vi "Vision_Left_R2.0.vi"() -> ()   [LabVIEW 2015]
uses:
  <vilib>/vision/Pattern Matching.llb/IMAQ Curve Parameters.ctl
  <vilib>/vision/Pattern Matching.llb/IMAQ Match Range Setting.ctl
panel:
  out "Current Correlation":sgl
  in  "Correlation Score Threshold":sgl
  out "New Min Score":dbl=879.6385864257812
  out "New Low Scale":dbl=38.665856552124026
  out "New high Scale":dbl=79.77148170471192
  in  "Absolute\nMinimum Score":dbl=800.0
  in  "Absolute\nMaximum Scale":dbl=300.0
  in  "Absolute\nMinimum Scale":dbl=10.0
  in  "Score Decay \nFactor":dbl=50.0
  in  "ROI_factor(Horiztonal) (4 b)":sgl=5.0
  in  "ROI_factor(vertical) (4 b)":sgl=1.5
  in  "ROI_factor(vertical) (5 b)":sgl=2.7
  in  "ROI_factor(Horiztonal) (5 b)":sgl=4.7
  in  "ROI_factor(Horiztonal) (2 b)":sgl=1.5
  in  "ROI_factor(vertical) (2 b)":sgl=2.5
  in  "Minimum Score\nSub 2":dbl=950.0
  in  "Minimum Score\nSub 3":dbl=900.0
  in  "Minimum Score\nSub 4":dbl=850.0
  in  "Minimum Score\nNormal 5":dbl=800.0
  in  "ROBOT STATE\n(fwd, bwd, neither)":i32
  out "Scale \nCushion":dbl=20.552812576293945
  in  "Score\nCushion":dbl=150.0
  in  "Default No Lock\nSetting Values":T1={"Min Scale"=20.0, "Max Scale"=170.0, "Min Score"=800.0}
  out "Next Template":T2(ring)
  in  "4 / 3\nTransition Scale":sgl=85.0
  in  "5 / 4\nTransition Scale":sgl=60.0
  in  "3 / 2\nTransition Scale":sgl=100.0
  in  "Avg Scale - Last":dbl=59.21866912841797
  in  "Avg Score - Last":dbl=954.6385864257812
  in  "Max Window\n for Avg":u8=5
  in  "Valid Treshold\nfor Lock":i16=3
  out "Current  Score":sgl=951.2561
  out "Current  Scale":sgl=59.269463
  out "Current Valid?":bool
  out "Beacon - Scales":sgl[](array[numeric])=[0.0, 59.087868, 59.67315, 57.828133, 55.61106]
  out "beacon - Scores":sgl[](array[numeric])=[0.0, 997.01117, 999.39996, 999.517, 998.72253]
  out "Beacons Found":bool[](array[boolean])=[FALSE, TRUE, TRUE, TRUE, TRUE]
  in  "Horiztonall Beacon \nCushion (pixels)":sgl=20.0
  in  "Sub - 4 - FIle Path":path=path "/home/lvuser/natinst/bin/BeaconTemplates/4_beacons_left.png"
  in  "Sub - 2 File Path":path=path "/home/lvuser/natinst/bin/BeaconTemplates/2_beacons_left.png"
  in  "Sub Beacon Template File Path - ARRAY":path[](array[path])=[path "/home/lvuser/natinst/bin/BeaconTemplates/Sub1.png", path "/home/lvuser/natinst/bin/BeaconTemplates/Sub2.png", path "/home/lvuser/natinst/bin/BeaconTemplates/Sub3.png", path "/home/lvuser/natinst/bin/BeaconTemplates/Sub4.png", path "/home/lvuser/natinst/bin/BeaconTemplates/Sub5.png"]
  in  "Sub - 3 - FIle Path":path=path "/home/lvuser/natinst/bin/BeaconTemplates/3_beacons_left.png"
  in  "Normal - 5 - File Path":path=path "/home/lvuser/natinst/bin/BeaconTemplates/5_beacons.png"
  out "Tracking Info":T3={"Tracking Coordinates"={"X"=154.8973846435547, "Y"=87.84130859375}, "Current Valid"=TRUE, "Current State - Out"=enum."Sub - 2", "Setting Values"={"Min Score"=950.0, "Min Scale"=103.51155548095704, "Max Scale"=214.8787582397461}}
  out "Current Template":T2(ring)
  in  "Initial Template":T2(ring)
  out "dT":u32=1105
  out "Avg Scale":dbl=159.2824279785156
  out "Avg Score":dbl=995.22490234375
  out "Current Search Settings":T6={"Curve Parameters"={"Extraction Mode"=1, "Edge Threshold"=150, "Edge Filter Size"=0, "Min Length"=15, "Row Search Step Size"=10, "Col Search Step Size"=10, "Max Endpoint Gap"=2, "Closed"=TRUE, "Subpixel"=TRUE}, "Match Mode"={"Rotation"=FALSE, "Scale"=TRUE, "Occlusion"=TRUE, "Reserved"=FALSE, "Reserved"=FALSE, "Reserved"=FALSE}, "Range Settings"=[{"Match Constraints"=0, "Min"=-2.0, "Max"=2.0}, {"Match Constraints"=1, "Min"=103.59702987670897, "Max"=214.96782608032225}, {"Match Constraints"=2, "Min"=0.0, "Max"=20.0}], "Number of Matches"=1, "Minimum Match Score"=950.0, "SubPixel Accuracy"=TRUE, "Adv. Geometric Match Options 2"=[{"Setup Data Item"=20, "Item Value"=0.0}, {"Setup Data Item"=22, "Item Value"=1.0}]} {"Curve Parameters"."Extraction Mode" items=["Normal", "Uniform Regions"]; "Curve Parameters"."Edge Filter Size" items=["Fine", "Normal", "Contour Tracing"]; "Curve Parameters"."Max Endpoint Gap" min=0; "Curve Parameters"."Col Search Step Size" min=1 max=255 step=1; "Curve Parameters"."Row Search Step Size" min=1 max=255 step=1; "Curve Parameters"."Min Length" min=0; "Curve Parameters"."Edge Threshold" min=1 max=350 step=1; "Range Settings"."Max" format="%.2f"; "Range Settings"."Min" format="%.2f"; "Range Settings"."Match Constraints" items=["Rotation Angle (degrees)", "Scale Factor (%)", "Occlusion (%)"]}
  out "Valid Scale History":dbl[](array[numeric])=[159.54193115234375, 159.0799560546875, 159.38912963867188, 159.05020141601562, 159.35092163085938, 159.10557556152344, 159.3151092529297, 159.3177947998047, 159.0937957763672, 159.64999389648438, 159.23023986816406, 159.07296752929688, 159.37905883789062, 156.36964416503906, 151.1900634765625, 132.892578125, 119.50423431396484, 108.0020523071289, 99.8529052734375, 93.15778350830078] format="%#_13g"
  out "Valid Score History":dbl[](array[numeric])=[995.82177734375, 997.0046997070312, 997.0046997070312, 997.0046997070312, 989.2886352539062, 997.0046997070312, 997.0046997070312, 996.4745483398438, 996.4745483398438, 995.4120483398438, 996.692138671875, 996.692138671875, 996.692138671875, 996.337890625, 998.2847290039062, 996.9906616210938, 1000.0, 999.7824096679688, 999.7824096679688, 999.7824096679688] format="%#_13g"
  out "Valid Beacon History - in":bool[](array[boolean])=[TRUE, TRUE, TRUE, TRUE, TRUE, TRUE, TRUE, TRUE, TRUE, TRUE, TRUE, TRUE, TRUE, TRUE, TRUE, TRUE, TRUE, TRUE, TRUE, TRUE]
  out "Startup Flag":bool
  out "Lock Status":bool
  out "Y Coordinates":sgl[](array[numeric])=[100.60873, 0.0, 0.0, 0.0, 0.0]
  out "X Coordinates":sgl[](array[numeric])=[108.138504, 0.0, 0.0, 0.0, 0.0]
  out "Right Image out":T7(plugin-control)
  in  "History Size":i32=20
  in  "INITIAL Search Settings":T6={"Curve Parameters"={"Extraction Mode"=1, "Edge Threshold"=150, "Edge Filter Size"=0, "Min Length"=15, "Row Search Step Size"=10, "Col Search Step Size"=10, "Max Endpoint Gap"=2, "Closed"=TRUE, "Subpixel"=TRUE}, "Match Mode"={"Rotation"=FALSE, "Scale"=TRUE, "Occlusion"=TRUE, "Reserved"=FALSE, "Reserved"=FALSE, "Reserved"=FALSE}, "Range Settings"=[{"Match Constraints"=0, "Min"=-2.0, "Max"=2.0}, {"Match Constraints"=1, "Min"=25.0, "Max"=100.0}, {"Match Constraints"=2, "Min"=0.0, "Max"=20.0}], "Number of Matches"=1, "Minimum Match Score"=800.0, "SubPixel Accuracy"=TRUE, "Adv. Geometric Match Options 2"=[{"Setup Data Item"=20, "Item Value"=0.0}, {"Setup Data Item"=22, "Item Value"=1.0}]} {"Curve Parameters"."Extraction Mode" items=["Normal", "Uniform Regions"]; "Curve Parameters"."Edge Filter Size" items=["Fine", "Normal", "Contour Tracing"]; "Curve Parameters"."Max Endpoint Gap" min=0; "Curve Parameters"."Col Search Step Size" min=1 max=255 step=1; "Curve Parameters"."Row Search Step Size" min=1 max=255 step=1; "Curve Parameters"."Min Length" min=0; "Curve Parameters"."Edge Threshold" min=1 max=350 step=1; "Range Settings"."Max" format="%.2f"; "Range Settings"."Min" format="%.2f"; "Range Settings"."Match Constraints" items=["Rotation Angle (degrees)", "Scale Factor (%)", "Occlusion (%)"]; "Adv. Geometric Match Options 2"."Setup Data Item" items=["Curve Extraction Mode", "Curve Edge Threshold", "Curve Edge Filter Size", "Min Curve Length", "Curve Row Search Step Size", "Curve Col Search Step Size", "Curve Max Endpoint Gap", "Extract Closed Curves", "Enable Subpixel Curve Extraction", "Enable Correlation Score", "Enable Subpixel Accuracy", "Subpixel Iterations", "Subpixel Tolerance", "Initial Match List Length", "Enable Target Template Curve Score", "Min Match Separation Distance", "Min Match Separation Angle", "Min Match Separation Scale", "Max Match Overlap", "Enable Coarse Result", "Enable Calibration Support", "Enable Contrast Reversal", "Search Strategy", "Refinement Match Factor", "Subpixel Match Factor"]}
  # "TEMPLATE FILE PATHS"
  # "Current Match Values"
  # "Range"
  # "Range"
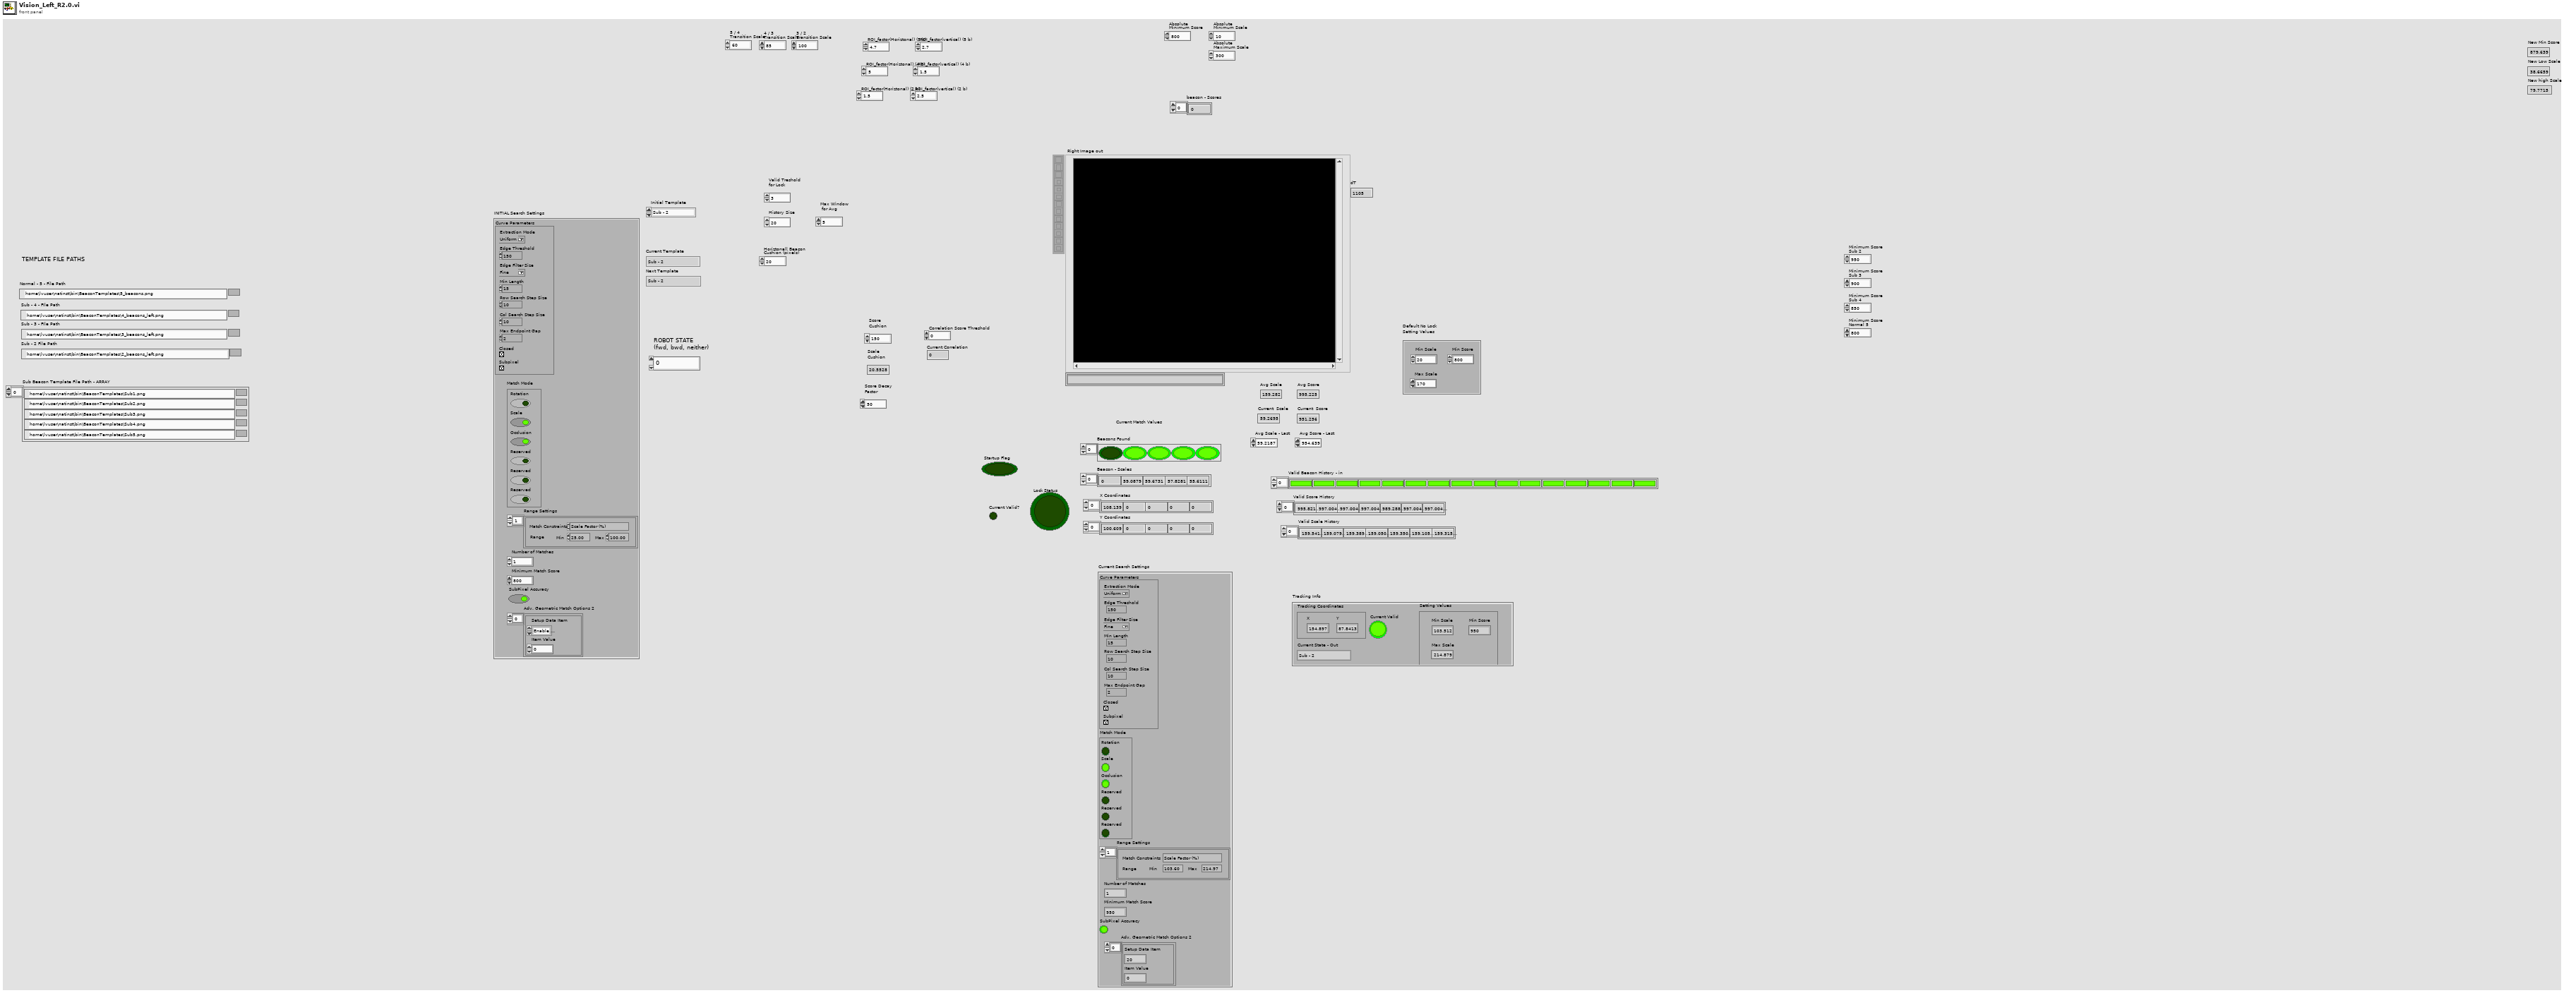
[diagram p1: front panel]
types:
  T1 = cluster{"Min Scale":dbl, "Max Scale":dbl, "Min Score":dbl}
  T2 = enum16{"Sub - 2", "Sub - 3", "Sub - 4", "Normal - 5"}
  T3 = cluster{"Tracking Coordinates":cluster{"X":dbl, "Y":dbl}, "Current Valid":bool, "Current State - Out":enum16{"Sub - 2", "Sub - 3", "Sub - 4", "Normal - 5"}, "Setting Values":cluster{"Min Score":dbl, "Min Scale":dbl, "Max Scale":dbl}}
  T4 = typedef "IMAQ Curve Parameters.ctl" = cluster{"Extraction Mode":u32, "Edge Threshold":i32, "Edge Filter Size":u32, "Min Length":i32, "Row Search Step Size":i32, "Col Search Step Size":i32, "Max Endpoint Gap":i32, "Closed":bool, "Subpixel":bool}
  T5 = typedef "IMAQ Match Range Setting.ctl" = cluster{"Match Constraints":u32, "Min":dbl, "Max":dbl}
  T6 = cluster{"Curve Parameters":T4, "Match Mode":cluster{"Rotation":bool, "Scale":bool, "Occlusion":bool, "Reserved":bool, "Reserved":bool, "Reserved":bool}, "Range Settings":T5[], "Number of Matches":i32, "Minimum Match Score":sgl, "SubPixel Accuracy":bool, "Adv. Geometric Match Options 2":cluster{"Setup Data Item":u16, "Item Value":dbl}[]}
  T7 = typedef "IMAQ Image.ctl" = refnum<image>
  T8 = typedef "Image Type" = u32
  T9 = typedef "ROI Descriptor" = cluster{"Global Rectangle":i32[], "Contours":cluster{"ID":enum32{"External", "Internal"}, "Type":u32, "Coordinates":i32[]}[]}
  T10 = typedef "IMAQ GM Match Report.ctl" = cluster{"Position":cluster{"x":sgl, "y":sgl}, "Angle":sgl, "Scale":sgl, "Score":sgl, "Bounding Box":cluster{"x":sgl, "y":sgl}[], "Contrast Reversed":bool, "Occlusion %":sgl, "Template Target Curve Score":sgl, "Target Template Curve Score":sgl, "Correlation Score":sgl}
  T11 = cluster{"Matches (Geometric Matching 1)[0]":T10, "Matches (Geometric Matching 1)[1]":T10, "Matches (Geometric Matching 1)[2]":T10, "Matches (Geometric Matching 1)[3]":T10, "Matches (Geometric Matching 1)[4]":T10, "Matches (Geometric Matching 1)[5]":T10, "Matches (Geometric Matching 1)[6]":T10, "Matches (Geometric Matching 1)[7]":T10, "Matches (Geometric Matching 1)[8]":T10}
  T12 = cluster{"Bounding Box[0]":cluster{"x":sgl, "y":sgl}, "Bounding Box[1]":cluster{"x":sgl, "y":sgl}, "Bounding Box[2]":cluster{"x":sgl, "y":sgl}, "Bounding Box[3]":cluster{"x":sgl, "y":sgl}, "Bounding Box[4]":cluster{"x":sgl, "y":sgl}, "Bounding Box[5]":cluster{"x":sgl, "y":sgl}, "Bounding Box[6]":cluster{"x":sgl, "y":sgl}, "Bounding Box[7]":cluster{"x":sgl, "y":sgl}, "Bounding Box[8]":cluster{"x":sgl, "y":sgl}}
  T13 = cluster{"Tracking Coordinates":cluster{"X":dbl, "Y":dbl}, "Current Valid":bool, "Current State - Out":enum16{"Sub - 2", "Sub - 3", "Sub - 4", "Normal - 5"}, "Setting Values":cluster{"Min Scale":dbl, "Max Scale":dbl, "Min Score":dbl}}
  T14 = typedef "IMAQ Rectangle" = cluster{"Left":i32, "Top":i32, "Right":i32, "Bottom":i32, "Rotation":dbl}
  T15 = cluster{"Minimum Score\nNormal 5":dbl, "Min":dbl, "Max":dbl}
  T16 = cluster{"Position":cluster{"x":dbl, "y":dbl}, bool, "Next Template":enum16{"Sub - 2", "Sub - 3", "Sub - 4", "Normal - 5"}, cluster{"Minimum Score\nNormal 5":dbl, "Min":dbl, "Max":dbl}}
  T17 = cluster{"Position":cluster{"x":dbl, "y":dbl}, bool, "Current Template":enum16{"Sub - 2", "Sub - 3", "Sub - 4", "Normal - 5"}, cluster{"Minimum Score\nNormal 5":dbl, "Min":dbl, "Max":dbl}}
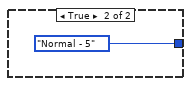
[diagram p3: hidden frame]
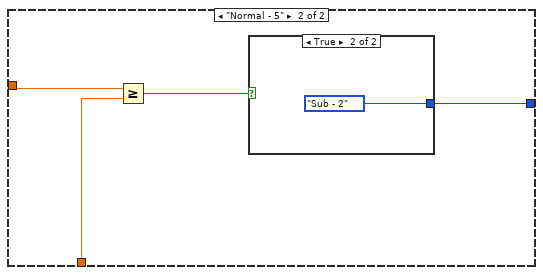
[diagram p4: hidden frame]
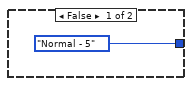
[diagram p5: hidden frame]
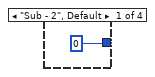
[diagram p7: hidden frame]
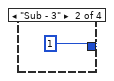
[diagram p8: hidden frame]
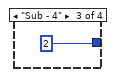
[diagram p9: hidden frame]
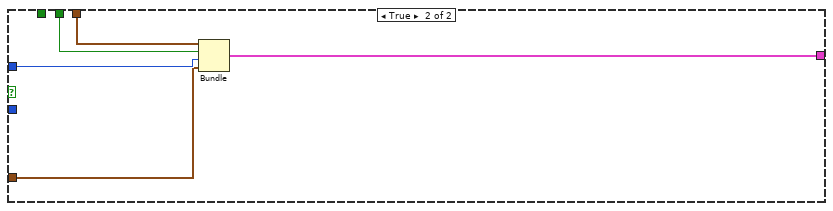
[diagram p10: hidden frame]
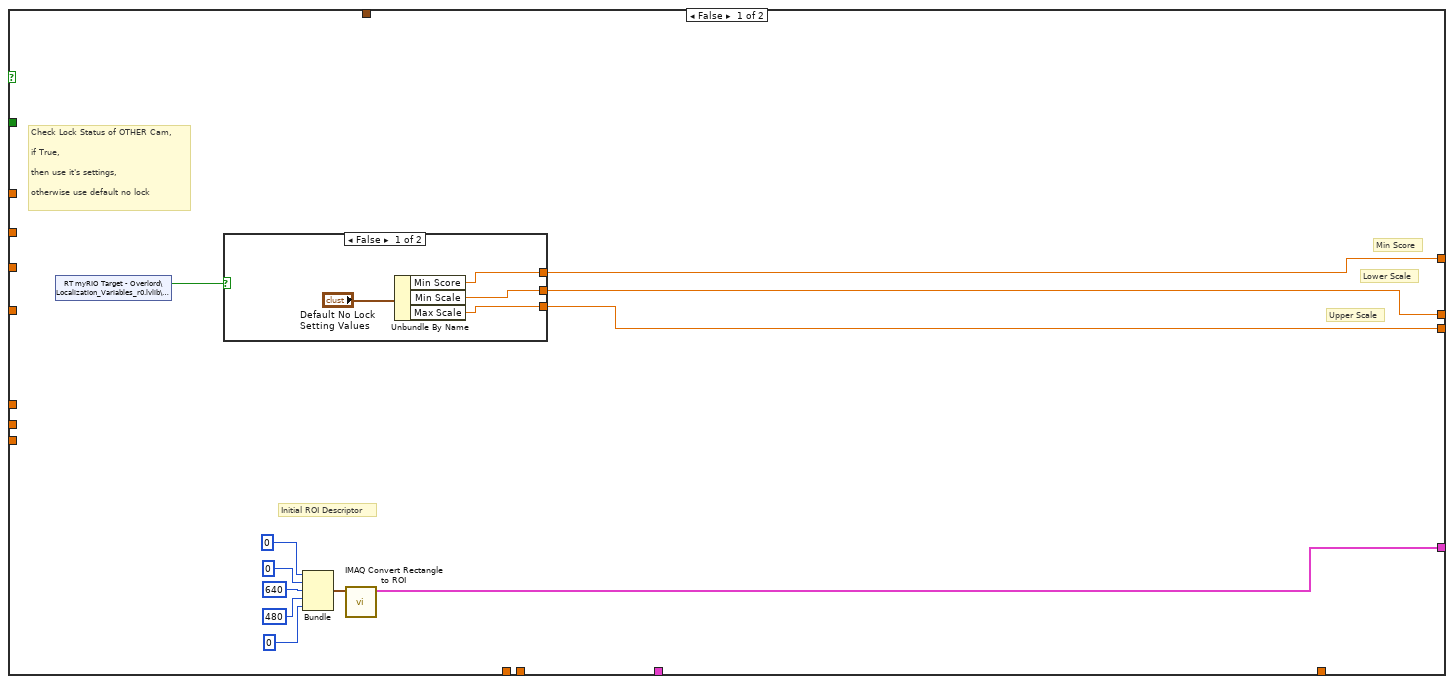
[diagram p13: hidden frame]
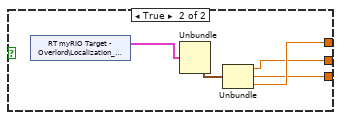
[diagram p14: hidden frame]
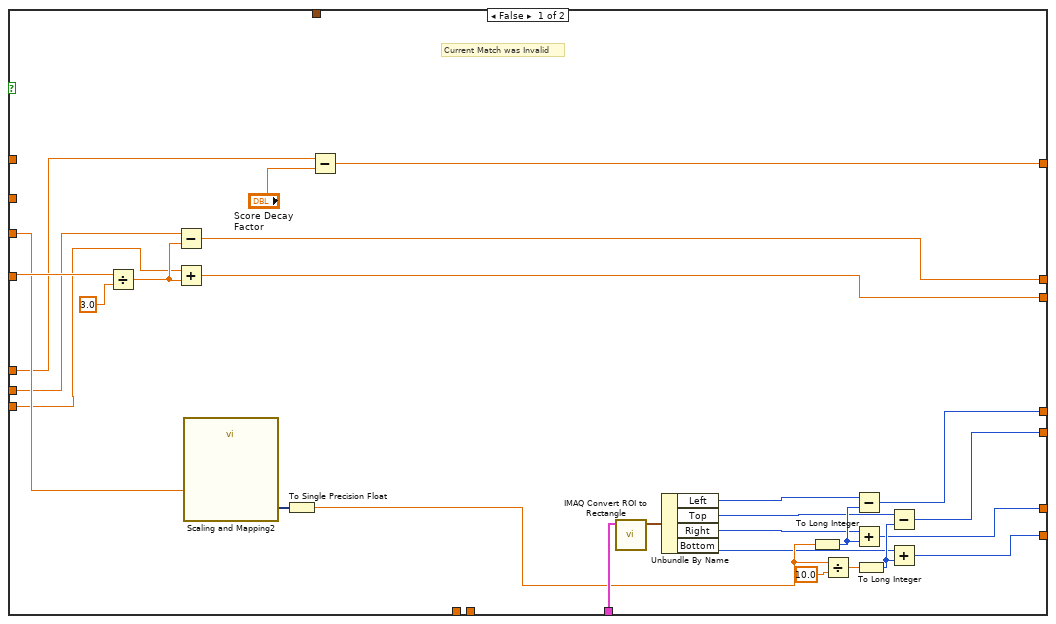
[diagram p15: hidden frame]
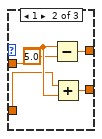
[diagram p16: hidden frame]
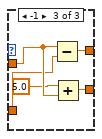
[diagram p17: hidden frame]
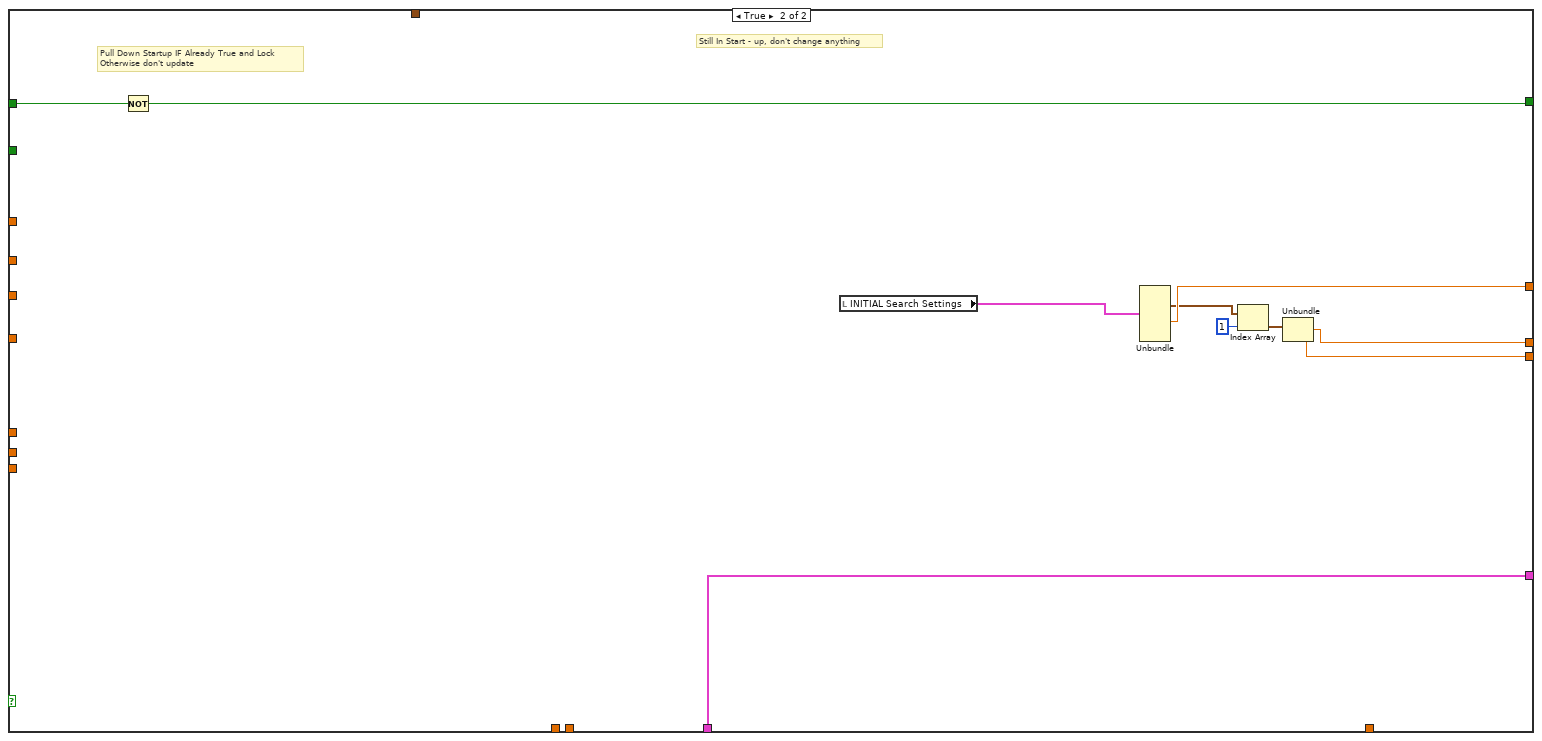
[diagram p18: hidden frame]
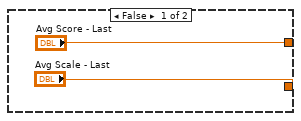
[diagram p19: hidden frame]
diagram:
  n1 = flat-sequence {
    tunnel: [w24] -> w12
    tunnel: ["INITIAL Search Settings"] -> w11
    tunnel: ["Initial Template"] -> w10
    tunnel: [TRUE] -> w9
    tunnel: [w21] -> w8
    tunnel: [w20] -> w7
    tunnel: [w19] -> w6
    tunnel: [w18] -> w5
    tunnel: [w17] -> w4
    tunnel: ["History Size"] -> w3
    tunnel: [750.0] -> w2
    tunnel: [100.0] -> w1
    tunnel: w12 -> [w46]
    tunnel: w11 -> [w45]
    tunnel: w10 -> [w44]
    tunnel: w9 -> [w43]
    tunnel: w8 -> [w39]
    tunnel: w7 -> [w36]
    tunnel: w6 -> [w42]
    tunnel: w5 -> [w41]
    tunnel: w4 -> [w40]
    tunnel: w3 -> [w38]
    tunnel: w2 -> [_]
    tunnel: w1 -> [_]
    frame #0 {
      w31 = T8 0 items=["Grayscale (U8)", "Grayscale (I16)", "Grayscale (SGL)", "Complex (CSG)", "RGB (U32)", "HSL (U32)", "RGB (U64)", "Grayscale (U16)"] ("Image Type")
      # "avg start scale"
      # "Score History"
      # "Scale History"
      # "Valid Match History\n(main beacon)"
      # "Template State"
      # "Search Parameters"
      # "StartUp = True"
      # "Initial ROI Descriptor"
      # "INITIALIZE"
      n2 = Bundle(0, 0, 640, 480, 0) -> (w30:cluster{i32, i32, i32, i32, i32})  [unwired: 1 in]
      n3 = call "IMAQ Convert Rectangle to ROI"("Rectangle"=w30) -> ("ROI Descriptor"=w24:T9)  [unwired: 8 in, 1 out]
      n4 = call "IMAQ Create"("Image Name"="Left_Image", "Image Type"=w31) -> ("New Image"=w21:T7, "error out"=w20:errorcluster)  [unwired: 3 in]
      n5 = Initialize Array(FALSE, "History Size") -> (w19:bool[])
      n6 = Initialize Array(0.0, "History Size") -> (w17:dbl[])
      n7 = Initialize Array(0.0, "History Size") -> (w18:dbl[])
    }
    frame #1 {
      # "Avg Scale"
      # "Avg Score"
      # "Score History"
      # "Scale History"
      # "Valid Match History\n(main beacon)"
      # "Sub Beacon Search Array"
      # "StartUp = True"
      # "Template State"
      # "Search Parameters"
      # "ROI"
      n8 = call "Tick Count"() -> ("Tick Count(mSec)"=w37:u32)
      n9 = while {
        shift-right: [w58] -> _
        shift-left: w46 -> [w65]
        shift-right: [w59] -> _
        shift-left: w45 -> [w66]
        shift-right: [w56] -> _
        shift-left: w44 -> [w74]
        shift-right: [w62] -> _
        shift-left: w43 -> [w64]
        shift-right: [w51] -> _
        shift-left: w42 -> [w52]
        shift-right: [w49] -> _
        shift-left: w41 -> [w50]
        shift-right: [w47] -> _
        shift-left: w40 -> [w48]
        shift-right: [w54] -> _
        shift-left: w39 -> [w67]
        tunnel: w38 -> [w72]
        shift-right: [w70] -> _
        shift-left: w37 -> [w71]
        tunnel: w36 -> [w53]
        stop <- FALSE stop-if-true
        n10 = call "Tick Count2"() -> ("Tick Count(mSec)"=w70:u32)
        n11 = Subtract(x=w70, y=w71) -> (x-y=→"dT":u32)
        n12 = flat-sequence {
          tunnel: [w81] -> w75
          tunnel: [w80] -> w73
          tunnel: [w79] -> w61
          tunnel: [w78] -> w68
          tunnel: w67 -> [w78]
          tunnel: [w78] -> w54
          tunnel: w53 -> [w77]
          tunnel: w75 -> [w195]
          tunnel: w74 -> [w95]
          tunnel: w73 -> [w100]
          tunnel: w52 -> [w176]
          tunnel: w50 -> [w175]
          tunnel: w48 -> [w174]
          tunnel: w72 -> [_]
          tunnel: w68 -> [w189]
          tunnel: w66 -> [w119]
          tunnel: w65 -> [w142]
          tunnel: w64 -> [w159]
          tunnel: [w118] -> w63
          tunnel: [w114] -> w62
          tunnel: w61 -> [w103]
          tunnel: [w103] -> w60
          tunnel: [w102] -> w57
          tunnel: [w101] -> w55
          tunnel: [w98] -> w51
          tunnel: [w97] -> w49
          tunnel: [w96] -> w47
          tunnel: w63 -> [w589]
          tunnel: w60 -> [w590]
          tunnel: [w589] -> w59
          tunnel: [w588] -> w58
          tunnel: w57 -> [w588]
          tunnel: [w587] -> w56
          tunnel: w55 -> [w587]
          frame #0 {
            # "Aquire Image"
            n13 = shared-variable "RT myRIO Target - Overlord\\Localization_Variables_r0.lvlib\\Left Servo Angle_Current"() -> (w79:dbl)  [unwired: 1 in, 1 out]
            n14 = call "Camera Acquisition"("error in"=w77) -> ("Image Out"=w81:T7, "error out"=w80:errorcluster)  [unwired: 24 in, 1 out]
          }
          frame #1 {
            w122 = u32 1 ("index")
            # "Current Template"
            # "Check if Next Template == Current TEmplate"
            # "Update Tracking Coordinates"
            # "Next Settings"
            # "Current Settings"
            # "Current Min\n& Max Scale"
            # "Scale"
            # "Min Score"
            # "Lower Scale"
            # "Upper Scale"
            # "Min Score out"
            # "Choose ROI Factor based on Next State"
            # "Avg Scale"
            # "Avg Score"
            # "StartUp Flag"
            # "Current Valid"
            # "image Lock"
            # "Update Search Settings"
            # "Image Lock?"
            # "Update Template"
            # "Score History"
            # "Min Required to use avarage"
            # "Scale History"
            # "History Size"
            # "Calculate Average Score/Scale"
            # "****# of previous in history that must be true\nin order for position to be considered \"locked\""
            # "Scale History"
            # "Score History"
            # "Valid History"
            # "Update History Data"
            # "1 Match FOund?"
            # "# of Sub Beacons"
            # "Sub Beacons to Search For"
            # "# Sub Beacons to Find in\norder to be valid"
            # "Template Filepath"
            # "Select Current Template Config"
            # "Pattern Match to Current Template"
            # "Apply FIltering"
            n15 = call "Camera - Filtering"("Image In"=w195, "Image Dst"=w189, "error in"=w100) -> ("Image Out"=w190:T7, "error out"=w99:errorcluster)  [unwired: 23 in]
            n16 = case shown="\"Normal - 5\"" w95 {
              tunnel: "Normal - 5 - File Path" -> [_ _ _ w586]
              tunnel: "Sub - 4 - FIle Path" -> [_ _ w581 _]
              tunnel: "Sub - 3 - FIle Path" -> [_ w575 _ _]
              tunnel: "Sub - 2 File Path" -> [w569 _ _ _]
              tunnel: [w569 w575 w581 w586] -> w188
              tunnel: [1 2 3 3] -> w178
              tunnel: [w567 w572 w578 w583] -> w183
              tunnel: [sgl 2.0 sgl 3.0 sgl 4.0 sgl 5.0] -> w184
              frame "Sub - 2", Default {
                w565 = FALSE
                w566 = TRUE
                n17 = Build Array(w566, w566, w565, w565, w565) -> (w567:bool[])
              }
              frame "Sub - 3" {
                w571 = FALSE
                w573 = TRUE
                n18 = Build Array(w573, w573, w573, w571, w571) -> (w572:bool[])
              }
              frame "Sub - 4" {
                w579 = TRUE
                n19 = Build Array(w579, w579, w579, w579, FALSE) -> (w578:bool[])
              }
              frame "Normal - 5" {
                (unwired) FALSE
                w584 = TRUE
                n20 = Build Array(w584, w584, w584, w584, w584) -> (w583:bool[])
              }
            }
            n21 = call "Geometric Pattern Matching"("Image In"=w190, "Image Dst"=w189, "ROI Descriptor (Geometric Matching 1)"=w142, "Settings (Geometric Matching 1)"=w119, "Template File Path (Geometric Matching 1)"=w188, "error in"=w99) -> ("Image Out"=w185:T7, "Matches (Geometric Matching 1)"=w86:T10[], "Number of Matches (Geometric Matching 1)"=w187:i32, "error out"=w182:errorcluster)  [unwired: 18 in]
            n22 = Array To Cluster(array=w86) -> (cluster=w87:T11)
            n23 = Unbundle By Name(w87) -> ("Matches (Geometric Matching 1)[0].Correlation Score"=w85:sgl)
            "Current Correlation" <- w85
            n24 = Equal?(x=w187, y=1) -> (x = y?=w89:bool)
            n25 = Greater?(x=w85, y="Correlation Score Threshold") -> (0:w88:bool)
            n26 = And(x=w89, y=w88) -> (x .and. y?=w90:bool)
            n27 = case shown="True" w90 {
              tunnel: w86 -> [_ w512]
              tunnel: w185 -> [w468 w491]
              tunnel: w184 -> [_ w506]
              tunnel: w183 -> [_ w493]
              tunnel: w182 -> [_ w490]
              tunnel: w119 -> [_ w488]
              tunnel: [w473 w486] -> w107
              tunnel: [w472 w485] -> w106
              tunnel: [w472 w484] -> w105
              tunnel: [w472 w483] -> w104
              tunnel: [w472 w482] -> w179
              tunnel: [w471 w481] -> w173
              tunnel: [w471 w480] -> w172
              tunnel: [w468 w479] -> w117
              tunnel: [w469 w478] -> w82
              frame False {
                w470 = 0.0
                w471 = sgl 0.0 ("Scale")
                n28 = Bundle(w470, w470) -> (w469:cluster{dbl, dbl})  [unwired: 1 in]
                n29 = Initialize Array(FALSE, 5 ("dimension size")) -> (w473:bool[])
                n30 = Initialize Array(0.0, 5 ("dimension size")) -> (w472:dbl[])
              }
              frame True {
                # "Build ROI for Individual Beacons Based on Main Bounding Box"
                # "Starting X Lower Bound"
                # "Beacons to Search For"
                # "Length of\nIndividual Beacon ROI"
                # "Length of Bounding Box"
                # "Draw Bounding Box on Display Image"
                n31 = Array To Cluster(array=w512) -> (cluster=w513:T11)
                n32 = Unbundle By Name(w513) -> ("Matches (Geometric Matching 1)[0].Position"=w478:cluster{"x":sgl, "y":sgl}, "Matches (Geometric Matching 1)[0].Bounding Box"=w510:cluster{"x":sgl, "y":sgl}[], "Matches (Geometric Matching 1)[0].Scale"=w481:sgl, "Matches (Geometric Matching 1)[0].Score"=w480:sgl)
                n33 = Array To Cluster(array=w510) -> (cluster=w511:T12)
                n34 = Unbundle By Name(w511) -> ("Bounding Box[0].x"=w504:sgl, "Bounding Box[0].y"=w500:sgl, "Bounding Box[2].x"=w507:sgl, "Bounding Box[2].y"=w499:sgl)
                n35 = Bundle("x"=w504, "y"=w500, "x"=w507, "y"=w499) -> (w509:cluster{"x":sgl, "y":sgl, "x":sgl, "y":sgl})  [unwired: 1 in]
                n36 = call "IMAQ Overlay Rectangle"("Rectangle"=w509, "Image"=w491) -> ("Image Out"=w487:T7)  [unwired: 8 in, 1 out]
                n37 = Subtract(x=w507, y=w504) -> (x-y=w508:sgl)
                n38 = Divide(x=w508, y=w506) -> (x/y=w505:sgl)
                n39 = Multiply(x="Horiztonall Beacon \nCushion (pixels)", y=w481) -> (x*y=w501:sgl)
                n40 = Divide(x=w501, y=sgl 100.0) -> (x/y=w496:sgl)
                n41 = Subtract(x=w500, y=w496) -> (x-y=w498:sgl)
                n42 = Add(x=w499, y=w496) -> (x+y=w497:sgl)
                n43 = for {
                  N: 5 -> [_]
                  tunnel: w493 -> [w559] mode=indexing
                  shift-right: [w553] -> _
                  shift-left: w504 -> [w558]
                  tunnel: w505 -> [w557]
                  tunnel: w498 -> [w550]
                  tunnel: w497 -> [w549]
                  tunnel: [w556] -> w492 mode=indexing
                  tunnel: w496 -> [w551]
                  # "Divide Bounding Box"
                  # "Upper Bound of Current is\nLower Bound for Next"
                  n44 = case shown="True" w559 {
                    tunnel: w558 -> [w560 w561]
                    tunnel: w557 -> [_ w563]
                    tunnel: [w560 w562] -> w553
                    tunnel: [w560 w561] -> w555
                    frame False {
                      # "Don't Care"
                    }
                    frame True {
                      # "X Lower Bound"
                      n45 = Add(x=w561, y=w563) -> (x+y=w562:sgl)
                    }
                  }
                  n46 = Subtract(x=w555, y=w551) -> (x-y=w554:sgl)
                  n47 = Add(x=w553, y=w551) -> (x+y=w552:sgl)
                  n48 = call "Bound_RO_R_R0I.vi"("Bottom Right - Y"=w549, "Right - X"=w552, "Top Left - Y"=w550, "Top  Left - x"=w554) -> ("ROI Descriptor"=w556:T9)  [unwired: 7 in]
                }
                n49 = for {
                  N: 5 -> [_]
                  tunnel: w491 -> [w526]
                  tunnel: w490 -> [w525]
                  tunnel: w492 -> [w518] mode=indexing
                  tunnel: "Sub Beacon Template File Path - ARRAY" -> [w524] mode=indexing
                  tunnel: [w523] -> w485 mode=indexing
                  tunnel: [w522] -> w484 mode=indexing
                  tunnel: [w521] -> w486 mode=indexing
                  tunnel: w493 -> [w520] mode=indexing
                  tunnel: w488 -> [w519]
                  shift-right: [w516] -> w479
                  shift-left: w487 -> [w517]
                  tunnel: [w515] -> w483 mode=indexing
                  tunnel: [w514] -> w482 mode=indexing
                  n50 = case shown="True" w520 {
                    tunnel: w526 -> [_ w541]
                    tunnel: w525 -> [_ w540]
                    tunnel: w518 -> [_ w539]
                    tunnel: w524 -> [_ w538]
                    tunnel: [w527 w534] -> w523
                    tunnel: [w527 w533] -> w522
                    tunnel: [FALSE w532] -> w521
                    tunnel: w519 -> [_ w531]
                    tunnel: [w527 w530] -> w515
                    tunnel: [w527 w529] -> w514
                    frame False {
                      w527 = sgl 0.0 ("x")
                    }
                    frame True {
                      n51 = call "Sub Beacon Pattern Match"("Image In"=w541, "ROI Descriptor (Geometric Matching 1)"=w539, "Settings (Geometric Matching 1)"=w531, "Template File Path (Geometric Matching 1)"=w538, "error in"=w540) -> ("Matches (Geometric Matching 1)"=w535:T10[], "Number of Matches (Geometric Matching 1)"=w536:i32)  [unwired: 19 in, 2 out]
                      n52 = Equal?(x=w536, y=1) -> (x = y?=w532:bool)
                      n53 = case shown="True" w532 {
                        tunnel: w535 -> [_ w547]
                        tunnel: [w542 w546] -> w534
                        tunnel: [w542 w545] -> w533
                        tunnel: [w542 w544] -> w530
                        tunnel: [w542 w543] -> w529
                        frame False {
                          w542 = sgl 0.0 ("x")
                        }
                        frame True {
                          n54 = Array To Cluster(array=w547) -> (cluster=w548:T11)
                          n55 = Unbundle By Name(w548) -> ("Matches (Geometric Matching 1)[0].Position.x"=w546:sgl, "Matches (Geometric Matching 1)[0].Position.y"=w545:sgl, "Matches (Geometric Matching 1)[0].Scale"=w544:sgl, "Matches (Geometric Matching 1)[0].Score"=w543:sgl)
                        }
                      }
                    }
                  }
                  n56 = call "IMAQ Overlay ROI"("ROI Descriptor"=w518, "Image"=w517) -> ("Image Out"=w516:T7)  [unwired: 8 in, 1 out]
                }
              }
            }
            "Beacons Found" <- w107
            "X Coordinates" <- w106
            "Y Coordinates" <- w105
            "Beacon - Scales" <- w104
            "beacon - Scores" <- w179
            "Current  Scale" <- w173
            "Current  Score" <- w172
            n57 = shared-variable "RT myRIO Target - Overlord\\Localization_Variables_r0.lvlib\\LEFT_BEACON_BOOL_array"(w107) -> ()  [unwired: 1 in, 1 out]
            n58 = shared-variable "RT myRIO Target - Overlord\\Localization_Variables_r0.lvlib\\LEFT_BEACON_X_array"(w106) -> ()  [unwired: 1 in, 1 out]
            n59 = shared-variable "RT myRIO Target - Overlord\\Localization_Variables_r0.lvlib\\LEFT_BEACON_Y_array"(w105) -> ()  [unwired: 1 in, 1 out]
            n60 = shared-variable "RT myRIO Target - Overlord\\Localization_Variables_r0.lvlib\\LEFT_BEACON_Scales"(w104) -> ()  [unwired: 1 in, 1 out]
            n61 = Boolean To (0,1)(Boolean=w107) -> (0, 1=w181:i16[])
            n62 = Add Array Elements(numeric array=w181) -> (sum=w180:i16)
            n63 = Greater Or Equal?(x=w180, y=w178) -> (x >= y?=w83:bool)
            "Current Valid?" <- w83
            n64 = local read "History Size"() -> (w164:i32)
            n65 = Decrement(x=w164) -> (x-1=w177:i32)
            n66 = for {
              N: w164 -> [_]
              shift-right: [w446] -> w98
              shift-left: w176 -> [w434]
              tunnel: w177 -> [w442]
              shift-right: [w439] -> w97
              shift-left: w175 -> [w441]
              shift-right: [w438] -> w96
              shift-left: w174 -> [w440]
              tunnel: w173 -> [w437]
              tunnel: w172 -> [w436]
              tunnel: w83 -> [w435]
              i -> [w445]
              # "Reverse Index"
              n67 = Subtract(x=w442, y=w445) -> (x-y=w443:i32)
              n68 = Equal To 0?(x=w443) -> (x = 0?=w444:bool)
              n69 = case shown="True" w444 {
                tunnel: w443 -> [w447 w466]
                tunnel: w434 -> [w457 w459]
                tunnel: [w455 w458] -> w446
                tunnel: w435 -> [_ w467]
                tunnel: w441 -> [w452 w465]
                tunnel: w440 -> [w451 w464]
                tunnel: [w450 w462] -> w439
                tunnel: [w449 w463] -> w438
                tunnel: w437 -> [_ w461]
                tunnel: w436 -> [_ w460]
                frame False {
                  # "Shift Old"
                  n70 = Decrement(x=w447) -> (x-1=w448:i32)
                  n71 = Index Array(array=w457, index=w448) -> (element=w456:bool)
                  n72 = Index Array(array=w452, index=w448) -> (element=w454:dbl)
                  n73 = Index Array(array=w451, index=w448) -> (element=w453:dbl)
                  n74 = Replace Array Subset(array=w457, new element=w456, index=w447) -> (w455:bool[])
                  n75 = Replace Array Subset(array=w452, new element=w454, index=w447) -> (w450:dbl[])
                  n76 = Replace Array Subset(array=w451, new element=w453, index=w447) -> (w449:dbl[])
                }
                frame True {
                  # "Score"
                  # "Scale"
                  # "Valid"
                  # "insert New"
                  n77 = Replace Array Subset(array=w465, new element=w461, index=w466) -> (w462:dbl[])
                  n78 = Replace Array Subset(array=w464, new element=w460, index=w466) -> (w463:dbl[])
                  n79 = Replace Array Subset(array=w459, new element=w467, index=w466) -> (w458:bool[])
                }
              }
            }
            n80 = Boolean To (0,1)(Boolean=w98) -> (0, 1=w170:i16[])
            n81 = Add Array Elements(numeric array=w170) -> (sum=w169:i16)
            n82 = Greater Or Equal?(x=w169, y="Valid Treshold\nfor Lock") -> (x >= y?=w93:bool)
            "Lock Status" <- w93
            n83 = shared-variable "RT myRIO Target - Overlord\\Localization_Variables_r0.lvlib\\Image Lock - L"(w93) -> ()  [unwired: 1 in, 1 out]
            n84 = Initialize Array(u8 0, "Max Window\n for Avg") -> (w167:u8[])
            n85 = while {
              shift-right: [w417] -> w163
              shift-left: w167 -> [w419]
              tunnel: w98 -> [w425] mode=indexing
              shift-right: [w423] -> w160
              shift-left: u8 0 -> [w426]
              tunnel: w164 -> [w424]
              tunnel: "Max Window\n for Avg" -> [w416]
              i -> [w418]
              stop <- w420 stop-if-true
              # "Grab Last 'X' Valid Indexes"
              n86 = case shown="True" w425 {
                tunnel: w426 -> [w428 w430]
                tunnel: [w428 w433] -> w423
                tunnel: w419 -> [w427 w432]
                tunnel: w418 -> [_ w431]
                tunnel: [w427 w429] -> w417
                frame False {
                }
                frame True {
                  # "Update Index\nto use"
                  # "Increment\nValid Count"
                  n87 = Replace Array Subset(array=w432, new element=w431, index=w430) -> (w429:u8[])
                  n88 = Increment(x=w430) -> (x+1=w433:u8)
                }
              }
              n89 = Greater?(x=w418, y=w424) -> (0:w421:bool)
              n90 = Greater Or Equal?(x=w423, y=w416) -> (x >= y?=w422:bool)
              n91 = Or(x=w422, y=w421) -> (x .or. y?=w420:bool)
            }
            n92 = Greater Or Equal?(x=w160, y=u8 2) -> (x >= y?=w161:bool)
            n93 = case shown="True" w161 {
              tunnel: w160 -> [_ w400]
              tunnel: w163 -> [_ w406]
              tunnel: w97 -> [_ w405]
              tunnel: w96 -> [_ w404]
              tunnel: ["Avg Score - Last" w398] -> w92
              tunnel: ["Avg Scale - Last" w397] -> w155
              frame False {
              }
              frame True {
                w403 = 0.0
                n94 = for {
                  N: w400 -> [_]
                  tunnel: w406 -> [w413] mode=indexing
                  tunnel: w405 -> [w415]
                  tunnel: w404 -> [w414]
                  shift-right: [w411] -> w402
                  shift-left: w403 -> [w409]
                  shift-right: [w412] -> w401
                  shift-left: w403 -> [w408]
                  # "Fetch Last Valid Values"
                  n95 = Index Array(array=w415, index=w413) -> (element=w410:dbl)
                  n96 = Index Array(array=w414, index=w413) -> (element=w407:dbl)
                  n97 = Add(x=w410, y=w409) -> (x+y=w411:dbl)
                  n98 = Add(x=w407, y=w408) -> (x+y=w412:dbl)
                }
                n99 = To Double Precision Float(number=w400) -> (double precision float=w399:dbl)
                n100 = Divide(x=w402, y=w399) -> (x/y=w398:dbl)
                n101 = Divide(x=w401, y=w399) -> (x/y=w397:dbl)
                n102 = local write "Avg Scale - Last"(w398) -> ()
                n103 = local write "Avg Score - Last"(w397) -> ()
              }
            }
            "Avg Score" <- w155
            "Avg Scale" <- w92
            n104 = case shown="True" w93 {
              tunnel: w95 -> [w196 w200]
              tunnel: "5 / 4\nTransition Scale" -> [_ w199]
              tunnel: w92 -> [_ w198]
              tunnel: [w196 w197] -> w91
              frame False {
              }
              frame True {
                n105 = case shown="\"Sub - 2\", Default" w200 {
                  tunnel: w199 -> [w203 w209]
                  tunnel: w198 -> [w204 w210]
                  tunnel: [w201 w207] -> w197
                  frame "Sub - 2", Default {
                    n106 = Less Or Equal?(x=w204, y=w203) -> (x <= y?=w202:bool)
                    n107 = case shown="False" w202 {
                      tunnel: [T2."Normal - 5" ("Initial Template") T2."Normal - 5" ("Initial Template")] -> w201
                      frame False {
                      }
                      frame True {
                      }
                    }
                  }
                  frame "Normal - 5" {
                    n108 = Greater Or Equal?(x=w210, y=w209) -> (x >= y?=w208:bool)
                    n109 = case shown="True" w208 {
                      tunnel: [T2."Normal - 5" ("Initial Template") T2."Sub - 2" ("Initial Template")] -> w207
                      frame False {
                      }
                      frame True {
                      }
                    }
                  }
                }
              }
            }
            "Next Template" <- w91
            n110 = call "Scaling and Mapping"("Signals"=w92) -> ("Scaled Signals"=w158:dynamicdata)  [unwired: 9 in, 1 out]
            n111 = Unbundle By Name(w119) -> ("Minimum Match Score"=w126:sgl, "Range Settings"=w123:T5[])
            n112 = To Single Precision Float(number=w158) -> (single precision float=w157:sgl)
            "Scale \nCushion" <- w157
            n113 = Index Array(array=w123, index=u32 1) -> (element=w127:T5)
            n114 = Unbundle(w127) -> ("Min"=w125:dbl, "Max"=w124:dbl)  [unwired: 1 out]
            n115 = case shown="\"Normal - 5\"" w91 {
              tunnel: "ROI_factor(vertical) (5 b)" -> [_ _ w260]
              tunnel: "ROI_factor(Horiztonal) (5 b)" -> [_ _ w259]
              tunnel: "ROI_factor(vertical) (4 b)" -> [_ w257 _]
              tunnel: "ROI_factor(Horiztonal) (4 b)" -> [_ w256 _]
              tunnel: "ROI_factor(vertical) (2 b)" -> [w254 _ _]
              tunnel: "ROI_factor(Horiztonal) (2 b)" -> [w253 _ _]
              tunnel: [w254 w257 w260] -> w145
              tunnel: [w253 w256 w259] -> w144
              tunnel: "Minimum Score\nSub 2" -> [w252 _ _]
              tunnel: [w252 w255 w258] -> w143
              tunnel: "Minimum Score\nNormal 5" -> [_ _ w258]
              tunnel: "Minimum Score\nSub 4" -> [_ w255 _]
              frame "Sub - 2" {
              }
              frame "Sub - 4", Default {
              }
              frame "Normal - 5" {
              }
            }
            n116 = case shown="False" w159 {
              tunnel: w93 -> [w279 w394]
              tunnel: [FALSE w393] -> w114
              tunnel: w83 -> [w278 _]
              tunnel: w157 -> [w274 _]
              tunnel: "Score\nCushion" -> [w276 _]
              tunnel: w155 -> [w277 _]
              tunnel: w92 -> [w275 _]
              tunnel: w145 -> [w273 _]
              tunnel: w144 -> [w272 _]
              tunnel: w143 -> [w271 _]
              tunnel: w142 -> [w270 w392]
              tunnel: [w269 w390] -> w131
              tunnel: [w268 w386] -> w130
              tunnel: [w267 w385] -> w129
              tunnel: [w266 w392] -> w102
              tunnel: w126 -> [w265 _]
              tunnel: w125 -> [w264 _]
              tunnel: w124 -> [w263 _]
              tunnel: w82 -> [w261 _]
              frame False {
                n117 = case shown="True" w279 {
                  tunnel: w278 -> [_ w322]
                  tunnel: w277 -> [_ w321]
                  tunnel: w276 -> [_ w320]
                  tunnel: w275 -> [_ w319]
                  tunnel: w274 -> [_ w318]
                  tunnel: w273 -> [_ w317]
                  tunnel: w272 -> [_ w316]
                  tunnel: w271 -> [_ w308]
                  tunnel: [w283 w310] -> w266
                  tunnel: [w282 w307] -> w269
                  tunnel: [w281 w306] -> w268
                  tunnel: [w280 w305] -> w267
                  tunnel: w270 -> [_ w304]
                  tunnel: w265 -> [_ w303]
                  tunnel: w264 -> [_ w302]
                  tunnel: w263 -> [_ w301]
                  tunnel: w261 -> [_ w300]
                  frame False {
                    # "Upper Scale"
                    # "Lower Scale"
                    # "Min Score"
                    # "Initial ROI Descriptor"
                    # "Check Lock Status of OTHER Cam,\n\nif True,\n\nthen use it's settings,\n\notherwise use default no lock"
                    n118 = shared-variable "RT myRIO Target - Overlord\\Localization_Variables_r0.lvlib\\Image Lock - R"() -> (w290:bool)  [unwired: 1 in, 1 out]
                    n119 = case shown="False" w290 {
                      tunnel: [w293 w297] -> w282
                      tunnel: [w291 w296] -> w280
                      tunnel: [w292 w295] -> w281
                      frame False {
                        n120 = Unbundle By Name("Default No Lock\nSetting Values") -> ("Min Score"=w293:dbl, "Min Scale"=w292:dbl, "Max Scale"=w291:dbl)
                      }
                      frame True {
                        n121 = shared-variable "RT myRIO Target - Overlord\\Localization_Variables_r0.lvlib\\Info - Right"() -> (w299:T13)  [unwired: 1 in, 1 out]
                        n122 = Unbundle(w299) -> ("Setting Values"=w298:T1)  [unwired: 3 out]
                        n123 = Unbundle(w298) -> ("Min Scale"=w295:dbl, "Max Scale"=w296:dbl, "Min Score"=w297:dbl)
                      }
                    }
                    n124 = Bundle(0, 0, 640, 480, 0) -> (w284:cluster{i32, i32, i32, i32, i32})  [unwired: 1 in]
                    n125 = call "IMAQ Convert Rectangle to ROI"("Rectangle"=w284) -> ("ROI Descriptor"=w283:T9)  [unwired: 8 in, 1 out]
                  }
                  frame True {
                    # "Apply Limit to Score"
                    # "Score out"
                    # "Apply Limits to ROI"
                    n126 = case shown="True" w322 {
                      tunnel: w321 -> [_ w369]
                      tunnel: w320 -> [_ w368]
                      tunnel: w319 -> [w342 w357]
                      tunnel: w318 -> [w349 w367]
                      tunnel: w317 -> [_ w362]
                      tunnel: w316 -> [_ w361]
                      tunnel: [w329 w360] -> w314
                      tunnel: [w328 w356] -> w313
                      tunnel: [w327 w359] -> w312
                      tunnel: [w326 w358] -> w311
                      tunnel: [w345 w355] -> w309
                      tunnel: [w344 w354] -> w306
                      tunnel: [w343 w353] -> w305
                      tunnel: w304 -> [w339 _]
                      tunnel: w303 -> [w325 _]
                      tunnel: w302 -> [w324 _]
                      tunnel: w301 -> [w323 _]
                      tunnel: w300 -> [_ w350]
                      frame False {
                        # "Current Match was Invalid"
                        n127 = Divide(x=w349, y=sgl 3.0) -> (x/y=w347:sgl)
                        n128 = Subtract(x=w324, y=w347) -> (x-y=w344:dbl)
                        n129 = Add(x=w323, y=w347) -> (x+y=w343:dbl)
                        n130 = call "Scaling and Mapping2"("Signals"=w342) -> ("Scaled Signals"=w341:dynamicdata)  [unwired: 9 in, 1 out]
                        n131 = To Single Precision Float(number=w341) -> (single precision float=w334:sgl)
                        n132 = Subtract(x=w325, y="Score Decay \nFactor") -> (x-y=w345:dbl)
                        n133 = call "IMAQ Convert ROI to Rectangle"("ROI Descriptor"=w339) -> ("Rectangle"=w340:T14)  [unwired: 8 in, 1 out]
                        n134 = Unbundle By Name(w340) -> ("Left"=w333:i32, "Top"=w332:i32, "Right"=w331:i32, "Bottom"=w330:i32)
                        n135 = To Long Integer(number=w334) -> (32bit integer=w336:i32)
                        n136 = Divide(x=w334, y=sgl 10.0) -> (x/y=w338:sgl)
                        n137 = Subtract(x=w333, y=w336) -> (x-y=w329:i32)
                        n138 = Add(x=w331, y=w336) -> (x+y=w327:i32)
                        n139 = To Long Integer(number=w338) -> (32bit integer=w335:i32)
                        n140 = Subtract(x=w332, y=w335) -> (x-y=w328:i32)
                        n141 = Add(x=w330, y=w335) -> (x+y=w326:i32)
                      }
                      frame True {
                        (unwired) sgl 109.0 ("x")
                        (unwired) sgl 159.0 ("x")
                        # "Current Match was Valid"
                        # "Center of Image"
                        # "Main ROI"
                        # "Horizontal Scale \n(smaller number = smaller ROI)"
                        n142 = Subtract(x=w369, y=w368) -> (x-y=w355:dbl)
                        n143 = case shown="0, Default" "ROBOT STATE\n(fwd, bwd, neither)" {
                          tunnel: w357 -> [w374 w379 w384]
                          tunnel: [w373 w375 w380] -> w353
                          tunnel: w367 -> [w371 w378 w383]
                          tunnel: [w372 w376 w381] -> w354
                          frame 0, Default {
                            n144 = Subtract(x=w374, y=w371) -> (x-y=w372:dbl)
                            n145 = Add(x=w371, y=w374) -> (x+y=w373:dbl)
                          }
                          frame 1 {
                            n146 = Subtract(x=w379, y=5.0) -> (x-y=w376:dbl)
                            n147 = Add(x=w378, y=w379) -> (x+y=w375:dbl)
                          }
                          frame -1 {
                            n148 = Subtract(x=w384, y=w383) -> (x-y=w381:dbl)
                            n149 = Add(x=5.0 ("y"), y=w384) -> (x+y=w380:dbl)
                          }
                        }
                        n150 = Unbundle(w350) -> ("x"=w352:dbl, "y"=w351:dbl)
                        n151 = Divide(x=w357, y=w362) -> (x/y=w365:dbl)
                        n152 = Multiply(x=w357, y=w361) -> (x*y=w363:dbl)
                        n153 = Divide(x=w363, y=sgl 2.0) -> (x/y=w366:dbl)
                        n154 = Add(x=w351, y=w365) -> (x+y=w358:dbl)
                        n155 = Subtract(x=w351, y=w365) -> (x-y=w356:dbl)
                        n156 = Subtract(x=w352, y=w366) -> (x-y=w360:dbl)
                        n157 = Add(x=w366, y=w352) -> (x+y=w359:dbl)
                      }
                    }
                    n158 = Greater?(x=w309, y=w308) -> (0:w315:bool)
                    n159 = call "Bound_RO_R_R0I.vi"("Bottom Right - Y"=w311, "Right - X"=w312, "Top Left - Y"=w313, "Top  Left - x"=w314) -> ("ROI Descriptor"=w310:T9)  [unwired: 7 in]
                    n160 = Select(t=w309, s=w315, f=w308) -> (s? t:f=w307:dbl)
                  }
                }
              }
              frame True {
                # "Pull Down Startup IF Already True and Lock\nOtherwise don't update"
                # "Still In Start - up, don't change anything"
                n161 = Not(x=w394) -> (.not. x?=w393:bool)
                n162 = local read "INITIAL Search Settings"() -> (w391:T6)
                n163 = Unbundle(w391) -> ("Range Settings"=w388:T5[], "Minimum Match Score"=w390:sgl)  [unwired: 5 out]
                n164 = Index Array(array=w388, index=1) -> (element=w387:T5)
                n165 = Unbundle(w387) -> ("Min"=w386:dbl, "Max"=w385:dbl)  [unwired: 1 out]
              }
            }
            n166 = call "IMAQ Overlay ROI"("ROI Descriptor"=w102, "Image"=w117) -> ("Image Out"=→"Right Image out":T7)  [unwired: 8 in, 1 out]
            n167 = Less?(x=w131, y="Absolute\nMinimum Score") -> (x < y?=w135:bool)
            n168 = Less?(x=w130, y="Absolute\nMinimum Scale") -> (x < y?=w138:bool)
            n169 = Greater?(x=w129, y="Absolute\nMaximum Scale") -> (0:w141:bool)
            n170 = Greater?(x=w130, y=w129) -> (0:w137:bool)
            n171 = Less?(x=w129, y=w130) -> (x < y?=w140:bool)
            n172 = Select(t="Absolute\nMinimum Score", s=w135, f=w131) -> (s? t:f=w113:dbl)
            "New Min Score" <- w113
            n173 = Or(x=w138, y=w137) -> (x .or. y?=w136:bool)
            n174 = Or(x=w141, y=w140) -> (x .or. y?=w139:bool)
            n175 = Select(t="Absolute\nMinimum Scale", s=w136, f=w130) -> (s? t:f=w112:dbl)
            "New Low Scale" <- w112
            n176 = Select(t="Absolute\nMaximum Scale", s=w139, f=w129) -> (s? t:f=w111:dbl)
            "New high Scale" <- w111
            n177 = Bundle("index"=w122, "Min"=w112, "Max"=w111) -> (w121:cluster{"index":u32, "Min":dbl, "Max":dbl})  [unwired: 1 in]
            n178 = Replace Array Subset(array=w123, new element=w121, index=w122) -> (w120:T5[])
            n179 = Bundle By Name(cluster=w119, "Minimum Match Score"=w113, "Range Settings"=w120) -> (w118:T6)
            n180 = local read "Current Template"() -> (w115:T2)
            n181 = local read "Next Template"() -> (w101:T2)
            n182 = Equal?(x=w115, y=w101) -> (x = y?=w116:bool)
            n183 = Bundle("Minimum Score\nNormal 5"=w113, "Min"=w112, "Max"=w111) -> (w110:T15)  [unwired: 1 in]
            n184 = case shown="False" w116 {
              tunnel: w115 -> [_ w249]
              tunnel: w82 -> [w221 w251]
              tunnel: w83 -> [w214 w250]
              tunnel: [w213 w248] -> w109
              tunnel: w107 -> [w222 _]
              tunnel: w110 -> [w217 w247]
              tunnel: w101 -> [w215 _]
              frame False {
                # "Check if Tracking is Available for the Next Template State"
                n185 = case shown="\"Normal - 5\"" w215 {
                  tunnel: [0 1 2 1] -> w220
                  frame "Sub - 2", Default {
                  }
                  frame "Sub - 3" {
                  }
                  frame "Sub - 4" {
                  }
                  frame "Normal - 5" {
                  }
                }
                n186 = Index Array(array=w222, index=w220) -> (element=w223:bool)
                n187 = local read "Y Coordinates"() -> (w218:sgl[])
                n188 = local read "X Coordinates"() -> (w219:sgl[])
                n189 = case shown="True" w223 {
                  tunnel: w219 -> [_ w242]
                  tunnel: w218 -> [_ w241]
                  tunnel: [w224 w238] -> w216
                  tunnel: w221 -> [w224 w239]
                  tunnel: w220 -> [_ w240]
                  frame False {
                  }
                  frame True {
                    w235 = sgl 0.4 ("y")
                    n190 = Unbundle(w239) -> ("x"=w236:dbl, "y"=w234:dbl)
                    n191 = Index Array(array=w242, index=w240) -> (element=w231:sgl)
                    n192 = Index Array(array=w241, index=w240) -> (element=w232:sgl)
                    n193 = Subtract(x=sgl 1.0, y=w235) -> (x-y=w233:sgl)
                    n194 = Multiply(x=w233, y=w231) -> (x*y=w229:sgl)
                    n195 = Multiply(x=w233, y=w232) -> (x*y=w227:sgl)
                    n196 = Multiply(x=w235, y=w236) -> (x*y=w230:dbl)
                    n197 = Multiply(x=w235, y=w234) -> (x*y=w228:dbl)
                    n198 = Add(x=w230, y=w229) -> (x+y=w226:dbl)
                    n199 = Add(x=w228, y=w227) -> (x+y=w225:dbl)
                    n200 = Bundle(w226, w225) -> (w238:cluster{dbl, dbl})  [unwired: 1 in]
                  }
                }
                n201 = Bundle("Position"=w216, w214, "Next Template"=w215, w217) -> (w213:T16)  [unwired: 1 in]
              }
              frame True {
                n202 = Bundle("Position"=w251, w250, "Current Template"=w249, w247) -> (w248:T17)  [unwired: 1 in]
              }
            }
            "Tracking Info" <- w109
            n203 = shared-variable "RT myRIO Target - Overlord\\Localization_Variables_r0.lvlib\\Info - Left"(w109) -> ()  [unwired: 1 in, 1 out]
          }
          frame #2 {
            n204 = shared-variable "RT myRIO Target - Overlord\\Localization_Variables_r0.lvlib\\Left Servo Angle_Image"(w590) -> ()  [unwired: 1 in, 1 out]
            n205 = shared-variable "RT myRIO Target - Overlord\\Localization_Variables_r0.lvlib\\Left_Flag"(TRUE ("RIGHT_FLAG")) -> ()  [unwired: 1 in, 1 out]
          }
        }
        "Startup Flag" <- w64
        "Valid Scale History" <- w50
        "Valid Beacon History - in" <- w52
        "Valid Score History" <- w48
        "Current Search Settings" <- w66
        "Current Template" <- w74
      }
    }
  }
